vi "Update.vi"(11 "Core Data in":T1) -> (2 "Screen":picture, 3 "Core Data out":T1)   [LabVIEW 2022 SP3, in "Application.lvlib"]
uses:
  Application.lvlib
  Core Data.ctl
  Scene/Scene.lvclass
  Mouse Button Held.ctl
  Scene/Scene.lvclass/Scene.ctl
  Scene/Transform And Project.vi
  Scene/Raster.vi
  Scene/Update Object.vi
  Scene/Update Transforms.vi
  Libraries/Utility/Convert Pixels To Picture.vi
  Present.vi/5bb89e80-4431-4a04-aab7-f6923ae8e18e.vi
  Present.vi/5002ab1c-b7b6-4038-93be-709e90c08d53.vi
  Draw Help.vi
  Draw Stats.vi
  Scene/Transform And Project.vi/196e4586-e654-41ec-a3a4-43fea5068e8e.vi
  Libraries/3D/Calculate View Matrix.vi
  Scene/Transform And Project.vi/a59a4b44-279f-4314-be75-e28f6a03f0ec.vi
  Transform And Project Single Object.vi
  Libraries/3D/Sort Triangles.vi
  Scene/Raster.vi/edb3f0c2-b950-4a44-8897-096d76b30880.vi
  Scene/Raster.vi/76d78098-f527-454b-a08a-aac5a717328f.vi
  Libraries/3D/Raster.vi
  Libraries/Utility/Convert Pixels To Picture.vi/d601d993-a776-4dc8-89c7-357d8398c88c.vi
  Libraries/Utility/Convert Pixels To Picture.vi/7816d0d6-8e4d-41a2-85ac-ed82f1435763.vi
  <vilib>/Utility/High Resolution Relative Seconds.vi
  Draw Help.vi/9f43915e-2be4-4177-985d-f5d8817b1a37.vi
  Libraries/Utility/Convert Seconds To Milliseconds.vi
  Sub Vs/Create Y Rotation Matrix.vi
  Libraries/3D/Multiply Vector By Matrix.vi
  Libraries/3D/Point At.vi
  Libraries/3D/Matrix Quick Invert.vi
  Libraries/3D/Normal.vi
  Libraries/3D/Project And Illuminate Triangle.vi
  Libraries/3D/Apply View Matrix.vi
  Libraries/3D/Transform Triangle.vi
  Sub Vs/Create Z Rotation Matrix.vi
  Sub Vs/Create X Rotation Matrix.vi
  Sub Vs/Create Translation Matrix.vi
  Libraries/3D/Check Raster Point In Range.vi
  Libraries/3D/Convert Point 2D (SGL) to Point 2D (I32).vi
  Libraries/Raster/Draw Triangle.vi
  Libraries/Raster/Draw Filled Triangle.vi
  Libraries/Raster/Clear Framebuffer.vi
  Libraries/3D/Degrees To Radians.vi
  Libraries/3D/Normalise Vector.vi
  Libraries/3D/Dot Product.vi
  Libraries/3D/Cross Product.vi
  Libraries/3D/Scale Point 3D (SGL) To Screen.vi
  Libraries/3D/Calculate Triangle Illumination.vi
  Libraries/Raster/Draw Line.vi
  Libraries/Raster/Draw Flat Bottom Filled Triangle.vi
  Libraries/Raster/Sort Points.vi
  Libraries/Raster/Draw Flat Top Filled Triangle.vi
  Libraries/Raster/Draw Line.vi/ce09c930-e75c-45b5-9de7-7d3097d91b09.vi
  Libraries/Raster/Draw Line.vi/8aa8c736-0805-475e-bbf3-9937bbefdeb4.vi
  Libraries/Raster/Draw Horizontal Line.vi
  Libraries/Raster/Draw Flat Bottom Filled Triangle.vi/c0c82237-b583-4fc1-b44f-40d02a28ecfd.vi
  Libraries/Raster/Draw Flat Bottom Filled Triangle.vi/53435b12-820c-4aea-aec4-7de16a894549.vi
  <vilib>/picture/picture.llb/Draw Unflattened Pixmap.vi
  <vilib>/picture/picture.llb/Draw True-Color Pixmap.vi
  <vilib>/picture/picture.llb/Get Text Rect.vi
  <vilib>/picture/picture.llb/Draw Text in Rect.vi
  Libraries/Utility/Measure Frame Rate.vi
  <vilib>/ptbypt/Probability & Statistics.llb/Mean PtByPt.vi
  <vilib>/Utility/colorconv.llb/Color to RGB.vi
  <vilib>/Utility/colorconv.llb/RGB to Color.vi
  <userlib>/_OpenG.lib/array/array.llb/Sort Array__ogtk.vi
  <userlib>/_OpenG.lib/array/array.llb/Sort 1D Array (SGL)__ogtk.vi
  <userlib>/_OpenG.lib/array/array.llb/Sort 1D Array (I32)__ogtk.vi
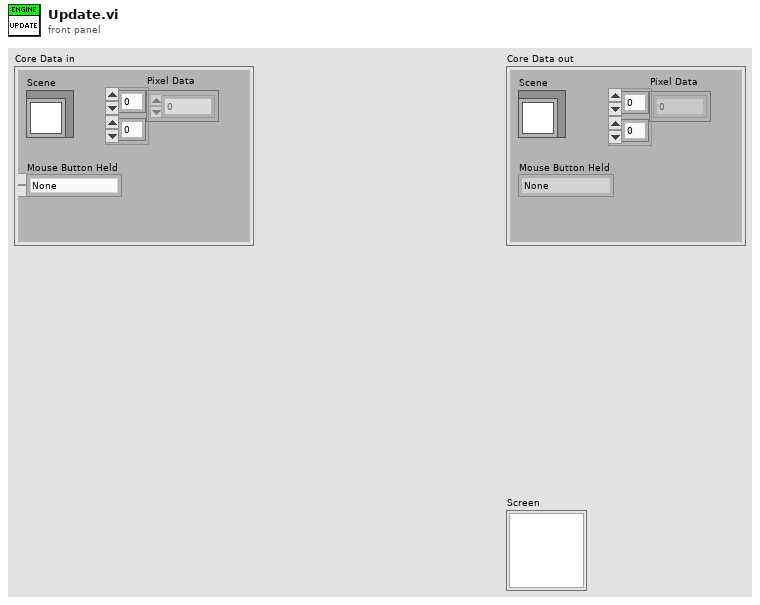
[diagram p1: front panel]
types:
  T1 = typedef "Application.lvlib/Core Data.ctl" = cluster{"Pixel Data":u32[][], "Scene":refnum<class "Scene.lvclass">, "Mouse Button Held":T2}
  T2 = typedef "Application.lvlib/Mouse Button Held.ctl" = enum16{"None", "Left", "Middle", "Right"}
  T3 = typedef "Application.lvlib/Scene.lvclass/Stats.ctl" = cluster{"Transform And Project Duration":dbl, "Raster Duration":dbl, "Present Duration":dbl, "Frame Rate":dbl, "Visible Triangles":i32, "Delta Time":dbl}
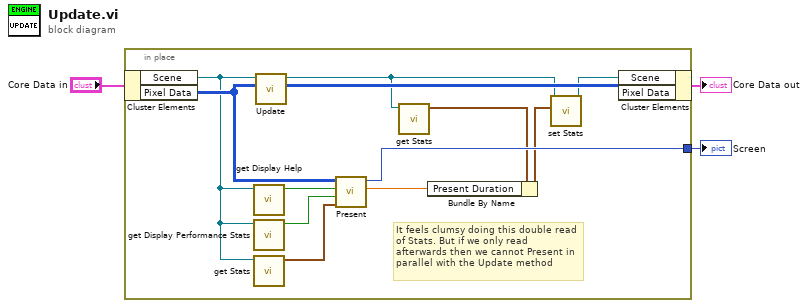
[diagram p0: block diagram]
diagram:
  n1 = in-place {
    in-place-border: [w13] -> w2
    # "It feels clumsy doing this double read of Stats. But if we only read afterwards then we cannot Present in parallel with the Update method"
    n2 = in-place-cluster #1("Core Data in") -> ("Scene"=w5:refnum<class "Scene.lvclass">, "Pixel Data"=w14:u32[][])
    n3 = call "get Display Help.vi"("Scene in"=w5) -> ("Display Help"=w7:bool)  [unwired: 10 in]
    n4 = call "get Display Performance Stats.vi"("Scene in"=w5) -> ("Display Stats"=w6:bool)  [unwired: 10 in]
    n5 = call "get Stats.vi"("Scene in"=w5) -> ("Stats"=w4:T3)  [unwired: 10 in]
    n6 = call "Update.vi"("Pixel Data in"=w14, "Scene in"=w5) -> ("Pixel Data out"=w15:u32[][], "Scene out"=w11:refnum<class "Scene.lvclass">)  [unwired: 8 in]
    n7 = call "Present.vi"("Stats"=w4, "Display Stats"=w6, "Display Help"=w7, "Pixel Data"=w14) -> ("Present Duration [s]"=w9:dbl, "2D Picture"=w13:picture)  [unwired: 6 in]
    n8 = call "get Stats.vi"("Scene in"=w11) -> ("Stats"=w10:T3)  [unwired: 10 in]
    n9 = Bundle By Name(cluster=w10, "Present Duration"=w9) -> (w8:T3)
    n10 = call "set Stats.vi"("Stats"=w8, "Scene in"=w11) -> ("Scene out"=w12:refnum<class "Scene.lvclass">)  [unwired: 9 in]
    n11 = in-place-cluster #1("Scene"=w12, "Pixel Data"=w15) -> (→"Core Data out":T1)
  }
  "Screen" <- w2
